vi "3ColorCautionLamp.vi"() -> ()   [LabVIEW 2015]
panel:
  out "number":u32
  out "appended array":bool[](array[boolean])
  out "YLDRMErrorOut":errorcluster
  out "YLDRMPortOut":refnum<visa-resource-name>
  in  "Tank":dbl(slide) scale=0.0..100.0
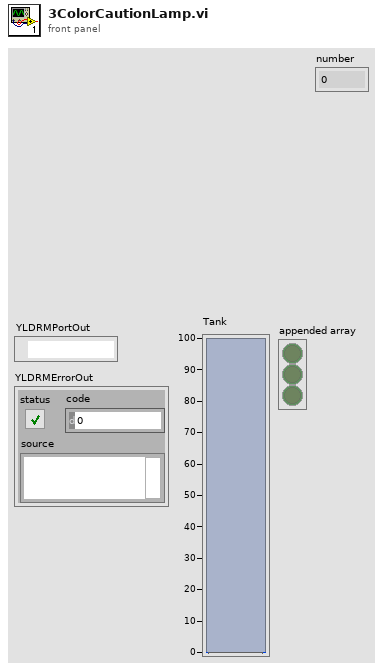
[diagram p1: front panel]
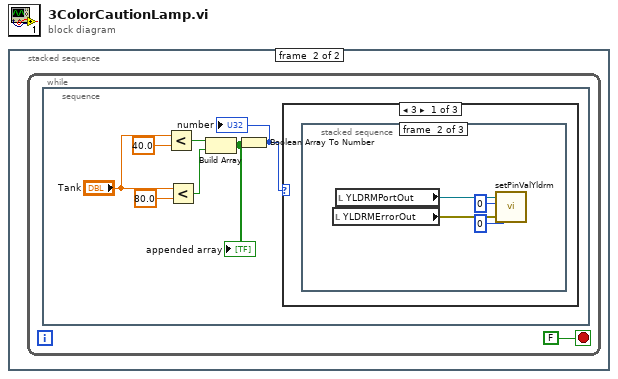
[diagram p0: block diagram]
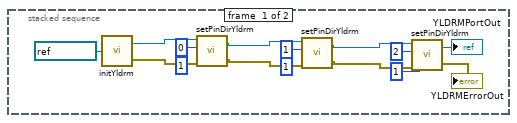
[diagram p2: hidden frame]
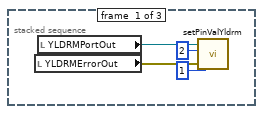
[diagram p3: hidden frame]
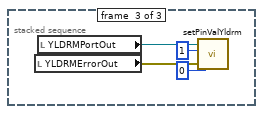
[diagram p4: hidden frame]
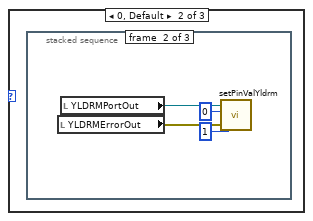
[diagram p5: hidden frame]
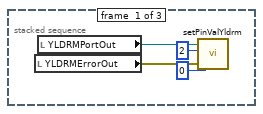
[diagram p6: hidden frame]
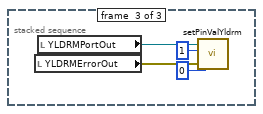
[diagram p7: hidden frame]
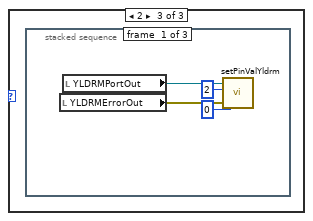
[diagram p8: hidden frame]
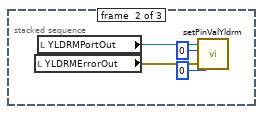
[diagram p9: hidden frame]
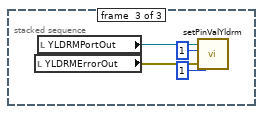
[diagram p10: hidden frame]
diagram:
  n1 = stacked-sequence {
    frame #0 {
      n2 = call "initYldrm.vi"("YLDRMPortInp"=refnum<visa-resource-name> "COM9") -> ("YLDRMPortOut"=w14:refnum<visa-resource-name>, "YLDRMErrorOut"=w13:errorcluster)
      n3 = call "setPinDirYldrm.vi"("YLDRMErrorInp"=w13, "dir"=u8 1, "pin"=u8 0, "YLDRMPortInp"=w14) -> ("YLDRMErrorOut"=w11:errorcluster, "YLDRMPortOut"=w12:refnum<visa-resource-name>)
      n4 = call "setPinDirYldrm.vi"("YLDRMErrorInp"=w11, "dir"=u8 1, "pin"=u8 1, "YLDRMPortInp"=w12) -> ("YLDRMErrorOut"=w9:errorcluster, "YLDRMPortOut"=w10:refnum<visa-resource-name>)
      n5 = call "setPinDirYldrm.vi"("YLDRMErrorInp"=w9, "dir"=u8 1, "pin"=u8 2, "YLDRMPortInp"=w10) -> ("YLDRMErrorOut"=→"YLDRMErrorOut":errorcluster, "YLDRMPortOut"=→"YLDRMPortOut":refnum<visa-resource-name>)
    }
    frame #1 {
      n6 = while {
        stop <- FALSE stop-if-true
        n7 = stacked-sequence {
          frame #0 {
            n8 = Less?(x="Tank", y=40.0) -> (x < y?=w20:bool)
            n9 = Less?(x="Tank", y=80.0) -> (x < y?=w19:bool)
            n10 = Build Array(w20, w19) -> (w18:bool[])
            "appended array" <- w18
            n11 = Boolean Array To Number(Boolean array=w18) -> (number=w17:u32)
            "number" <- w17
            n12 = case shown="3" w17 {
              frame 3 {
                n13 = stacked-sequence {
                  frame #0 {
                    n14 = local read "YLDRMErrorOut"() -> (w26:errorcluster)
                    n15 = local read "YLDRMPortOut"() -> (w27:refnum<visa-resource-name>)
                    n16 = call "setPinValYldrm.vi"("YLDRMErrorInp"=w26, "val"=u8 1, "pin"=u8 2, "YLDRMPortInp"=w27) -> ()  [unwired: 2 out]
                  }
                  frame #1 {
                    n17 = local read "YLDRMErrorOut"() -> (w30:errorcluster)
                    n18 = local read "YLDRMPortOut"() -> (w31:refnum<visa-resource-name>)
                    n19 = call "setPinValYldrm.vi"("YLDRMErrorInp"=w30, "val"=u8 0, "pin"=u8 0, "YLDRMPortInp"=w31) -> ()  [unwired: 2 out]
                  }
                  frame #2 {
                    n20 = local read "YLDRMErrorOut"() -> (w34:errorcluster)
                    n21 = local read "YLDRMPortOut"() -> (w35:refnum<visa-resource-name>)
                    n22 = call "setPinValYldrm.vi"("YLDRMErrorInp"=w34, "val"=u8 0, "pin"=u8 1, "YLDRMPortInp"=w35) -> ()  [unwired: 2 out]
                  }
                }
              }
              frame 0, Default {
                n23 = stacked-sequence {
                  frame #0 {
                    n24 = local read "YLDRMErrorOut"() -> (w38:errorcluster)
                    n25 = local read "YLDRMPortOut"() -> (w39:refnum<visa-resource-name>)
                    n26 = call "setPinValYldrm.vi"("YLDRMErrorInp"=w38, "val"=u8 0, "pin"=u8 2, "YLDRMPortInp"=w39) -> ()  [unwired: 2 out]
                  }
                  frame #1 {
                    n27 = local read "YLDRMErrorOut"() -> (w42:errorcluster)
                    n28 = local read "YLDRMPortOut"() -> (w43:refnum<visa-resource-name>)
                    n29 = call "setPinValYldrm.vi"("YLDRMErrorInp"=w42, "val"=u8 1, "pin"=u8 0, "YLDRMPortInp"=w43) -> ()  [unwired: 2 out]
                  }
                  frame #2 {
                    n30 = local read "YLDRMErrorOut"() -> (w46:errorcluster)
                    n31 = local read "YLDRMPortOut"() -> (w47:refnum<visa-resource-name>)
                    n32 = call "setPinValYldrm.vi"("YLDRMErrorInp"=w46, "val"=u8 0, "pin"=u8 1, "YLDRMPortInp"=w47) -> ()  [unwired: 2 out]
                  }
                }
              }
              frame 2 {
                n33 = stacked-sequence {
                  frame #0 {
                    n34 = local read "YLDRMErrorOut"() -> (w50:errorcluster)
                    n35 = local read "YLDRMPortOut"() -> (w51:refnum<visa-resource-name>)
                    n36 = call "setPinValYldrm.vi"("YLDRMErrorInp"=w50, "val"=u8 0, "pin"=u8 2, "YLDRMPortInp"=w51) -> ()  [unwired: 2 out]
                  }
                  frame #1 {
                    n37 = local read "YLDRMErrorOut"() -> (w54:errorcluster)
                    n38 = local read "YLDRMPortOut"() -> (w55:refnum<visa-resource-name>)
                    n39 = call "setPinValYldrm.vi"("YLDRMErrorInp"=w54, "val"=u8 0, "pin"=u8 0, "YLDRMPortInp"=w55) -> ()  [unwired: 2 out]
                  }
                  frame #2 {
                    n40 = local read "YLDRMErrorOut"() -> (w58:errorcluster)
                    n41 = local read "YLDRMPortOut"() -> (w59:refnum<visa-resource-name>)
                    n42 = call "setPinValYldrm.vi"("YLDRMErrorInp"=w58, "val"=u8 1, "pin"=u8 1, "YLDRMPortInp"=w59) -> ()  [unwired: 2 out]
                  }
                }
              }
            }
          }
        }
      }
    }
  }
